vi "Return Available Buffer.vi"(8 "error in (no error)":errorcluster, 10 "DMA Memory":refnum<data-value>, 11 "TDMS DAQ in":refnum<class "TDMS DAQ.lvclass">) -> (0 "error out":errorcluster, 3 "TDMS DAQ out":refnum<class "TDMS DAQ.lvclass">)   [LabVIEW 2025, in "TDMS DAQ.lvlib" / "TDMS DAQ.lvclass"]
uses:
  TDMS DAQ.lvclass
  TDMS DAQ.lvclass/TDMS DAQ.ctl
  DAQ Interface/DAQ Interface/DAQ Interface.lvclass
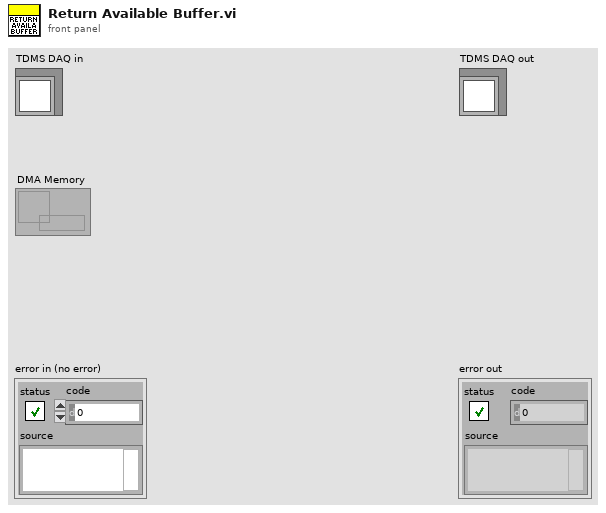
[diagram p1: front panel]
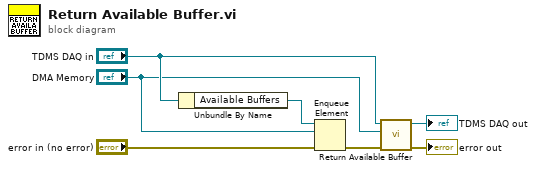
[diagram p0: block diagram]
diagram:
  n1 = Unbundle By Name("TDMS DAQ in") -> ("Available Buffers"=w4:refnum<queue>)
  n2 = Enqueue Element(queue=w4, element="DMA Memory", error in (no error)="error in (no error)") -> (error out=w1:errorcluster)  [unwired: 1 in, 2 out]
  n3 = call-parent "Return Available Buffer.vi"("error in (no error)"=w1, "DMA Memory"="DMA Memory", "DAQ Interface in"="TDMS DAQ in") -> ("error out"=→"error out":errorcluster, "DAQ Interface out"=→"TDMS DAQ out":refnum<class "TDMS DAQ.lvclass">)  [unwired: 7 in]
